vi "Update if Clear.vi"(8 "error in (no error)":errorcluster, 10 "Message Data":variant, 11 "Queue in":refnum<queue>) -> (0 "error out":errorcluster)   [LabVIEW 2018, in "Support Library.lvlib"]
uses:
  Support Library.lvlib
  Message Queue/Message Cluster.ctl
  Message Queue/Enqueue Message (Single).vi
  Message Queue/Message Queue.lvlib
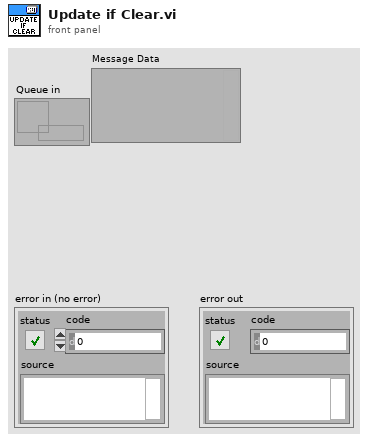
[diagram p1: front panel]
types:
  T1 = typedef "Support Library.lvlib/Message Queue.lvlib/Message Cluster.ctl" = cluster{"Message":string, "Message Data":variant}
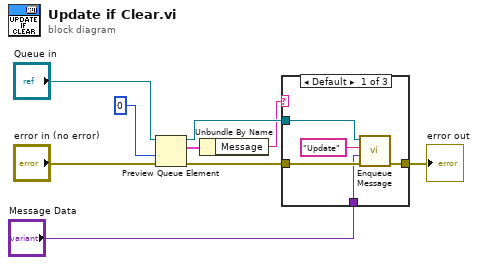
[diagram p0: block diagram]
diagram:
  n1 = Preview Queue Element(queue="Queue in", timeout in ms (-1)=0, error in (no error)="error in (no error)") -> (queue out=w5:refnum<queue>, element=w4:T1, error out=w2:errorcluster)  [unwired: 1 out]
  n2 = Unbundle By Name(w4) -> ("Message"=w3:string)
  n3 = case shown="Default" w3 {
    tunnel: w5 -> [w11 _ _]
    tunnel: [w12 w15 w16] -> w9
    tunnel: w2 -> [w13 w15 w16]
    tunnel: "Message Data" -> [w10 _ _]
    frame Default {
      n4 = call-poly "Enqueue Message.vi"("error in (no error)"=w13, "Message Data"=w10, "Message"="Update", "Message Queue"=w11) -> ("error out"=w12:errorcluster)  [unwired: 6 in, 1 out]
    }
    frame "Update" {
    }
    frame "Exit" {
    }
  }
  "error out" <- w9
